vi "Stop Core.vi"(10 "final error code":i32, 11 "CameraTesting in":refnum<class "CameraTesting.lvclass">) -> (3 "CameraTesting out":refnum<class "CameraTesting.lvclass">)   [LabVIEW 2020, in "CameraTesting.lvlib" / "CameraTesting.lvclass"]
doc: "(<B>Filename</B>: Actor Framework.lvlib:Actor.lvclass:Stop Core.vi)\n\nDefines what the actor does before it stops. Use the <B>final error code</B> input to determine whether the actor shut down in response to an error.\n\nBy default, this method passes the Stop message along to all auto-stop nested actors. A descendant class may override this method to define additional behavior, such as shutting down any processes the actor initiated in its override of the Actor Core method."
uses:
  CameraTesting.lvclass
  CameraTesting.lvclass/CameraTesting.ctl
  <vilib>/ActorFramework/Stop Msg/Stop Msg.lvclass/Stop Msg.ctl
  <vilib>/ActorFramework/Message Enqueuer/Message Enqueuer.lvclass/Message Enqueuer.ctl
  21e4e04d-f254-4266-b9ab-0eda022b0b68.vi
  <vilib>/ActorFramework/Stop Msg/Send Emergency Stop.vi
  <vilib>/ActorFramework/Stop Msg/Send Normal Stop.vi
  <vilib>/ActorFramework/Message Enqueuer/Enqueue Critical.vi
  <vilib>/ActorFramework/Message Enqueuer/Enqueue.vi
  <vilib>/ActorFramework/Stop Msg/Stop Msg.lvclass
  C:/Program Files (x86)/National Instruments/LabVIEW 2020/vi.lib/ActorFramework/Message/Message.lvclass
  <vilib>/ActorFramework/Message Priority Queue/Priority Enqueue.vi
  <vilib>/ActorFramework/Actor/Actor.lvclass
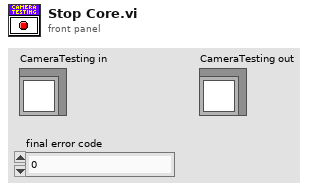
[diagram p1: front panel]
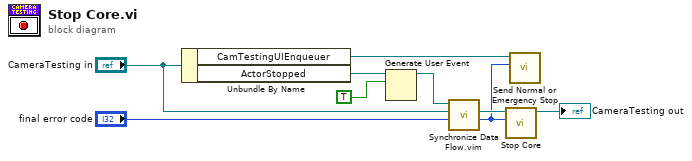
[diagram p0: block diagram]
diagram:
  n1 = Unbundle By Name("CameraTesting in") -> ("CamTestingUIEnqueuer"=w1:refnum<class "Message Enqueuer.lvclass">, "ActorStopped"=w8:refnum<user-event>)
  n2 = Generate User Event(user event=w8, event data cluster=TRUE ("event data")) -> (user event out=w6:refnum<user-event>)  [unwired: 2 in, 1 out]
  n3 = call "Synchronize Data Flow.vim"("input 3"="final error code", "input 2"="CameraTesting in", "input 1"=w6) -> ("output 3"=w2:i32, "output 2"=w3:refnum<class "CameraTesting.lvclass">)  [unwired: 1 in, 2 out]
  n4 = call-parent "Stop Core.vi"("final error code"=w2, "Actor in"=w3) -> ("Actor out"=→"CameraTesting out":refnum<class "CameraTesting.lvclass">)  [unwired: 9 in]
  n5 = call <vilib>:"Send Normal or Emergency Stop.vi"("final error code"=w2, "Message Enqueuer"=w1) -> ()  [unwired: 9 in, 1 out]
